vi "xmlCreate.vi"(1 "error in (no error)":errorcluster caption="错误输入（无错误）", 2 "XML file path":path caption="XML文件路径") -> (0 "error out":errorcluster caption="错误输出")   [LabVIEW 2011]
uses:
  <vilib>/xml/NI_XML.lvlib
  program files/worksoftware/Labview/resource/objmgr/DOMUserDefRef.rc
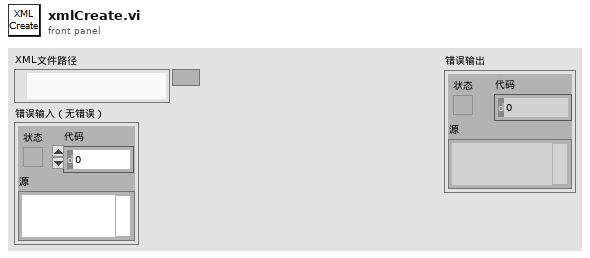
[diagram p1: front panel]
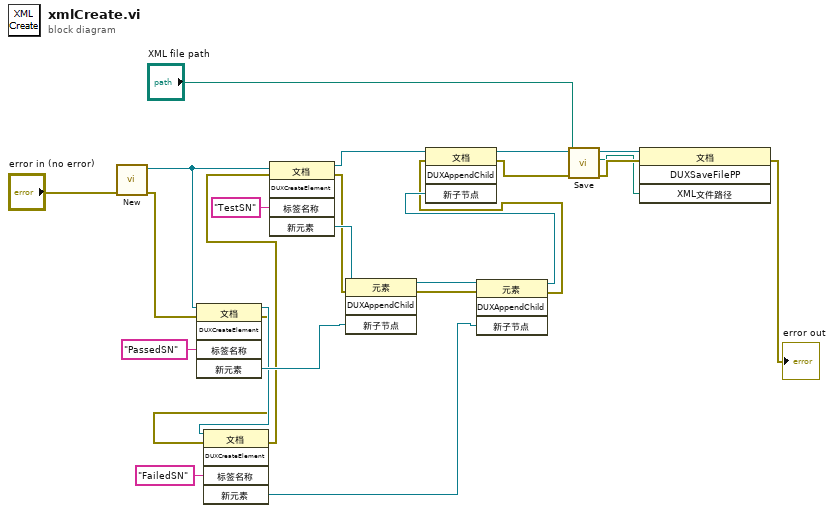
[diagram p0: block diagram]
diagram:
  n1 = call <vilib>:"New.vi"("error in (no error)"="error in (no error)") -> ("error out"=w12:errorcluster, "DOM document out"=w20:refnum<k20>)  [unwired: 7 in]
  n2 = invoke class="文档" method="DUXCreateElement"(reference=w20, error in=w12, "标签名称"="PassedSN") -> (reference out=w15:refnum<k20>, error out=w11:errorcluster, "新元素"=w17:refnum<k20>)  [unwired: 2 in, 2 out]
  n3 = invoke class="文档" method="DUXCreateElement"(reference=w15, error in=w11, "标签名称"="FailedSN") -> (error out=w10:errorcluster, "新元素"=w13:refnum<k20>)  [unwired: 2 in, 3 out]
  n4 = invoke class="文档" method="DUXCreateElement"(reference=w20, error in=w10, "标签名称"="TestSN") -> (reference out=w24:refnum<k20>, error out=w9:errorcluster, "新元素"=w21:refnum<k20>)  [unwired: 2 in, 2 out]
  n5 = invoke class="元素" method="DUXAppendChild"(reference=w21, error in=w9, "新子节点"=w17) -> (reference out=w18:refnum<k20>, error out=w8:errorcluster)  [unwired: 1 in, 2 out]
  n6 = invoke class="元素" method="DUXAppendChild"(reference=w18, error in=w8, "新子节点"=w13) -> (reference out=w16:refnum<k20>, error out=w7:errorcluster)  [unwired: 1 in, 2 out]
  n7 = invoke class="文档" method="DUXAppendChild"(reference=w24, error in=w7, "新子节点"=w16) -> (reference out=w23:refnum<k20>, error out=w6:errorcluster)  [unwired: 1 in, 2 out]
  n8 = call <vilib>:"Save.vi"("error in (no error)"=w6, "XML file path"="XML file path", "DOM document in"=w23) -> ("error out"=w3:errorcluster, "XML file path out"=w2:path, "DOM document out"=w4:refnum<k20>)  [unwired: 6 in]
  n9 = invoke class="文档" method="DUXSaveFilePP"(reference=w4, error in=w3, "XML文件路径"=w2) -> (error out=→"error out":errorcluster)  [unwired: 1 in, 3 out]
